vi "Read Position File.vi"(8 "error in (no error)":errorcluster, 11 "ViewableActor in":refnum<class "ViewableActor.lvclass">) -> (0 "error out":errorcluster, 3 "ViewableActor out":refnum<class "ViewableActor.lvclass">)   [LabVIEW 2014, in "ViewableActor.lvlib" / "ViewableActor.lvclass"]
uses:
  ViewableActor.lvclass
  ViewableActor.lvclass/ViewableActor.ctl
  Read Actor Name.vi
  Read SubPanel Ref.vi
  <vilib>/Utility/config.llb/Read Key (I32).vi
  <vilib>/Utility/config.llb/NI_LVConfig.lvlib
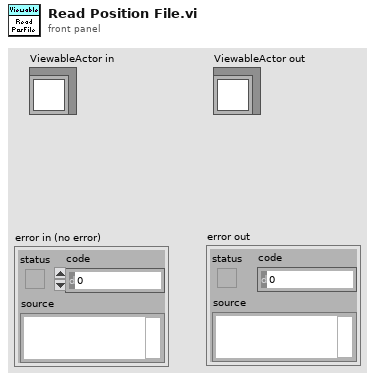
[diagram p1: front panel]
types:
  T1 = typedef "NI_LVConfig.lvlib/Config Data RefNum.ctl" = refnum<k1>
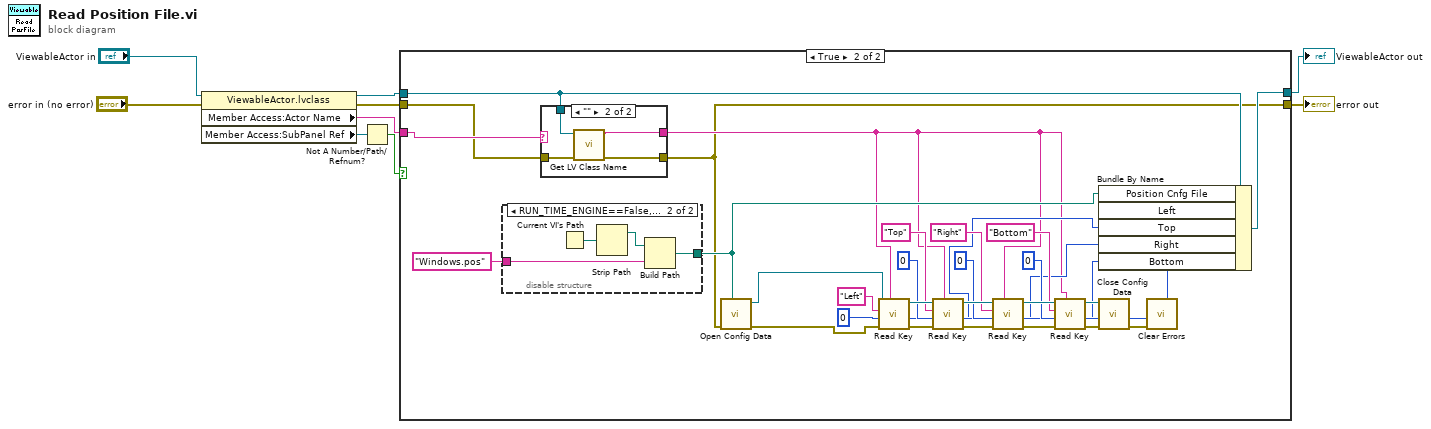
[diagram p0: block diagram]
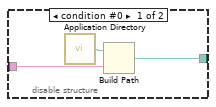
[diagram p4: hidden frame]
diagram:
  n1 = property class="ViewableActor.lvclass"(reference="ViewableActor in", error in="error in (no error)") -> (reference out=w5:refnum<class "ViewableActor.lvclass">, error out=w2:errorcluster, "Member Access:Actor Name"=w4:string, "Member Access:SubPanel Ref"=w7:refnum<vi>)
  n2 = Not A Number/Path/Refnum?(number/path/refnum=w7) -> (NaN/Path/Refnum?=w6:bool)
  n3 = case shown="True" w6 {
    tunnel: w5 -> [w11 w15]
    tunnel: [w11 w41] -> w9
    tunnel: w4 -> [_ w16]
    tunnel: w2 -> [w10 w13]
    tunnel: [w10 w12] -> w1
    frame False {
    }
    frame True {
      n4 = disable-structure shown="RUN_TIME_ENGINE==False, Default" {
        disable-tunnel: [w50 w52] -> w40
        disable-tunnel: "Windows.pos" ("string") -> [w49 w54]
        frame condition #0 {
          n5 = call <vilib>:"Application Directory.vi"() -> ("Application Directory"=w51:path)
          n6 = Build Path(base path=w51, name or relative path=w49) -> (appended path=w50:path)
        }
        frame condition #1 (active) {
          n7 = Current VI's Path() -> (path=w55:path)
          n8 = Strip Path(path=w55) -> (stripped path=w53:path)  [unwired: 1 out]
          n9 = Build Path(base path=w53, name or relative path=w54) -> (appended path=w52:path)
        }
      }
      n10 = case shown="\"\"" w16 {
        selector: w16 -> [w44 _]
        tunnel: w15 -> [_ w48]
        tunnel: [w44 w47] -> w14
        tunnel: w13 -> [w43 w46]
        tunnel: [w43 w45] -> w12
        frame Default {
        }
        frame "" {
          n11 = call <vilib>:"Get LV Class Name.vi"("error in (no error)"=w46, "object"=w48) -> ("error out"=w45:errorcluster, "class name"=w47:string)  [unwired: 8 in]
        }
      }
      n12 = call <vilib>:"Open Config Data.vi"("error in (no error)"=w12, "configuration file path"=w40) -> ("error out"=w38:errorcluster, "refnum"=w39:T1)  [unwired: 7 in, 1 out]
      n13 = call-poly <vilib>:"Read Key.vi"("section"=w14, "error in (no error)"=w38, "default value"=0, "key"="Left", "refnum"=w39) -> ("error out"=w36:errorcluster, "value"=w21:i32, "refnum out"=w37:T1)  [unwired: 3 in, 1 out]
      n14 = call-poly <vilib>:"Read Key.vi"("section"=w14, "error in (no error)"=w36, "default value"=0, "key"="Top", "refnum"=w37) -> ("error out"=w34:errorcluster, "value"=w20:i32, "refnum out"=w35:T1)  [unwired: 3 in, 1 out]
      n15 = call-poly <vilib>:"Read Key.vi"("section"=w14, "error in (no error)"=w34, "default value"=0, "key"="Right", "refnum"=w35) -> ("error out"=w32:errorcluster, "value"=w19:i32, "refnum out"=w33:T1)  [unwired: 3 in, 1 out]
      n16 = call-poly <vilib>:"Read Key.vi"("section"=w14, "error in (no error)"=w32, "default value"=0, "key"="Bottom", "refnum"=w33) -> ("error out"=w30:errorcluster, "value"=w18:i32, "refnum out"=w31:T1)  [unwired: 3 in, 1 out]
      n17 = Bundle By Name(cluster=w15, "Position Cnfg File"=w40, "Left"=w21, "Top"=w20, "Right"=w19, "Bottom"=w18) -> (w41:refnum<class "ViewableActor.lvclass">)
      n18 = call <vilib>:"Close Config Data.vi"("error in (no error)"=w30, "refnum"=w31) -> ("error out"=w17:errorcluster)  [unwired: 8 in, 1 out]
      n19 = call <vilib>:"Clear Errors.vi"("error in (no error)"=w17) -> ()  [unwired: 5 in, 2 out]
    }
  }
  "ViewableActor out" <- w9
  "error out" <- w1
